vi "Main.vi"(11 "_Rescript in":refnum<class "_Rescript.lvclass">) -> (0 "error out":errorcluster, 3 "_Rescript out":refnum<class "_Rescript.lvclass">)   [LabVIEW 2020, in "_Rescript.lvlib" / "_Rescript.lvclass"]
uses:
  _Rescript.lvclass
  _Rescript.lvclass/_Rescript.ctl
  _Shared/Name Specs/Name Specs.lvclass/Name Specs.ctl
  Actor/Actor/Actor.lvclass/Actor.ctl
  Msg/Msg/Msg.lvclass/Msg.ctl
  Actor/Actor/Actor.lvclass
  C:/git/jettl/src/jettl Tools/_Rescript/Type/Type.lvclass
  Msg/Msg/Msg.lvclass
  Type/Type.lvclass
  _Shared/Name Specs/Name Specs.lvclass
  Msg/Msg.lvlib
  Actor/Actor.lvlib
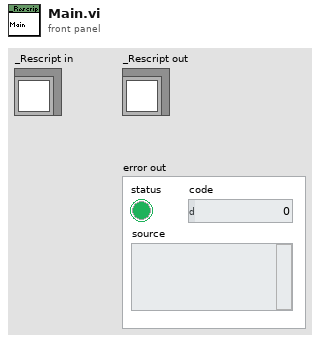
[diagram p1: front panel]
types:
  T1 = typedef "_Shared.lvlib/Name Stuff.ctl" = cluster{"Type (Enum)":T2, "Type (String)":string, "Name Library File Path":path, "Name":string, "Name Type":string}
  T2 = typedef "_Shared.lvlib/Type.ctl" = enum16{"Actor", "Msg"}
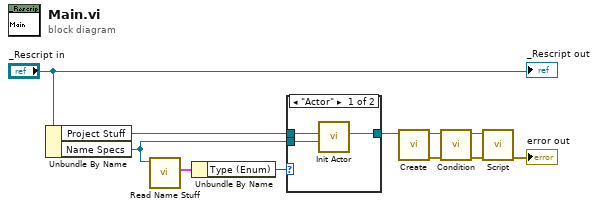
[diagram p0: block diagram]
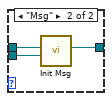
[diagram p2: hidden frame]
diagram:
  n1 = Unbundle By Name("_Rescript in") -> ("Project Stuff"=w2:refnum<class "Project Stuff.lvclass">, "Name Specs"=w1:refnum<class "Name Specs.lvclass">)
  n2 = call "Read Name Stuff.vi"("Name Specs in"=w1) -> ("Name Stuff"=w11:T1)  [unwired: 10 in]
  n3 = Unbundle By Name(w11) -> ("Type (Enum)"=w9:T2)
  n4 = case shown="\"Actor\"" w9 {
    tunnel: [w12 w17] -> w3
    tunnel: w2 -> [w14 w16]
    tunnel: w1 -> [w13 w15]
    frame "Actor" {
      n5 = call "Init Actor.vi"("Name Specs"=w13, "Project Stuff"=w14) -> ("Type"=w12:refnum<class "Type.lvclass">)  [unwired: 9 in]
    }
    frame "Msg" {
      n6 = call "Init Msg.vi"("Name Specs"=w15, "Project Stuff"=w16) -> ("Type"=w17:refnum<class "Type.lvclass">)  [unwired: 9 in]
    }
  }
  n7 = call-dynamic "Create.vi"("Type in"=w3) -> ("error out"=w6:errorcluster, "Type out"=w5:refnum<class "Type.lvclass">)  [unwired: 9 in]
  n8 = call-dynamic "Condition.vi"("error in"=w6, "Type in"=w5) -> ("error out"=w7:errorcluster, "Type out"=w4:refnum<class "Type.lvclass">)  [unwired: 8 in]
  n9 = call-dynamic "Script.vi"("error in"=w7, "Type in"=w4) -> ("error out"=→"error out":errorcluster)  [unwired: 8 in, 1 out]
  "_Rescript out" <- "_Rescript in"
